vi "质控测完标志全局 1.vi"() -> ()   [LabVIEW 2016, in "质控单元.lvlib"]
panel:
  in  "CODCr平行样测完标志":bool
  in  "CODCr加标回收测完标志":bool
  in  "CODCr质控流程中":bool
  in  "COD质控流程中":bool
  in  "总氮质控流程中":bool
  in  "总磷质控流程中":bool
  in  "氨氮质控流程中":bool
  in  "质控流程中":bool
  in  "总氮加标回收测完标志":bool
  in  "氨氮平行样测完标志":bool
  in  "氨氮加标回收测完标志":bool
  in  "COD加标回收测完标志":bool
  in  "总磷加标回收测完标志":bool
  in  "COD平行样测完标志":bool
  in  "总磷总氮平行样测完标志":bool
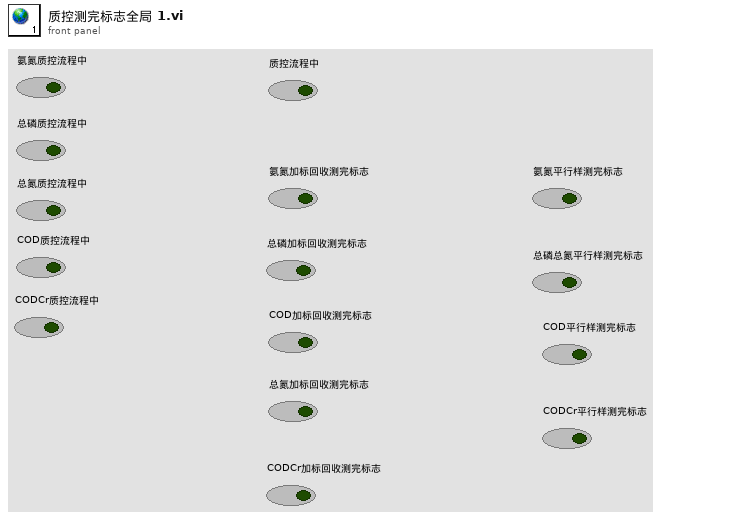
[diagram p1: front panel]
diagram:
